vi "Event.vi"() -> ()   [LabVIEW 2020]
panel:
  out "Gauge":dbl(knob) scale=0.0..10.0
  in  "Slide":dbl(slide) scale=0.0..10.0
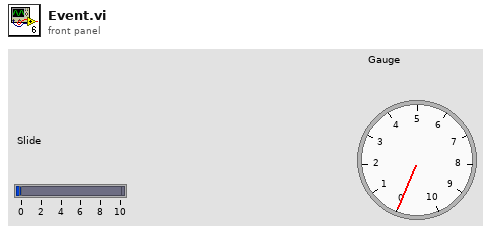
[diagram p1: front panel]
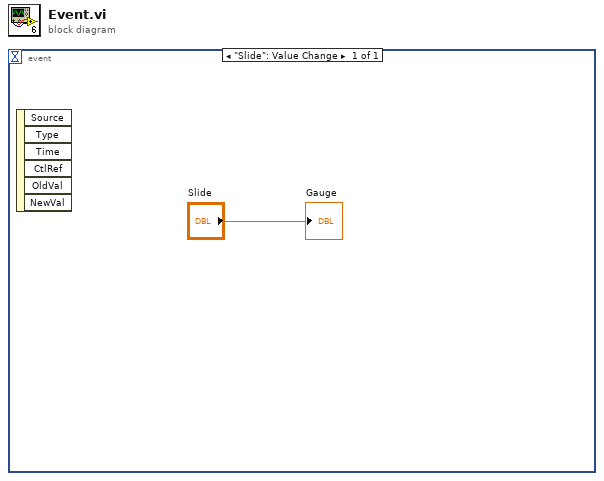
[diagram p0: block diagram]
diagram:
  n1 = event shown="[0] \"Slide\": Value Change" {
    selector: _ -> [_]
    dyn-events: _ -> [_]
    timeout: _ -> [_]
    event "Slide": Value Change {
      n2 = event-data() -> ()  [unwired: 1 in, 6 out]
      "Gauge" <- "Slide"
    }
  }
